vi "Conditionally Increment Data At Index.vi"(9 "Increment":bool, 10 "Data index":i32, 11 "Data in":dbl[](array[numeric])) -> (3 "Data out":dbl[](array[numeric]))   [LabVIEW 2019, in "NI Synchronization Engine.lvlib"]
uses:
  NI Synchronization Engine.lvlib
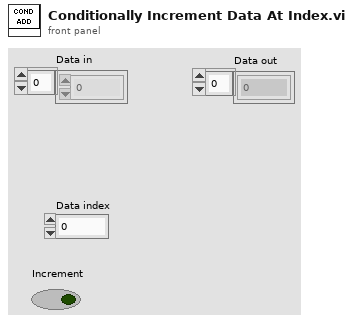
[diagram p1: front panel]
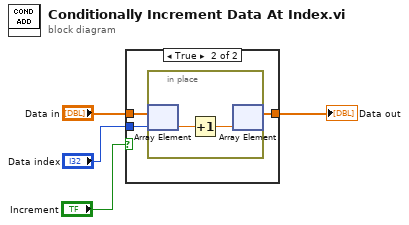
[diagram p0: block diagram]
diagram:
  n1 = case shown="True" "Increment" {
    tunnel: "Data in" -> [w5 w8]
    tunnel: "Data index" -> [_ w7]
    tunnel: [w5 w6] -> w2
    frame False {
    }
    frame True {
      n2 = in-place {
        n3 = in-place-array #1(w8, w7) -> (w10:dbl)
        n4 = Increment(x=w10) -> (x+1=w9:dbl)
        n5 = in-place-array #1(w9) -> (w6:dbl[])  [unwired: 1 out]
      }
    }
  }
  "Data out" <- w2
